vi "Read data.vi"(11 "communicator message in":refnum<class "communicator message.lvclass">) -> (3 "data":variant)   [LabVIEW 2015, in "communicator message.lvclass"]
uses:
  communicator message.lvclass
  communicator message.lvclass/communicator message.ctl
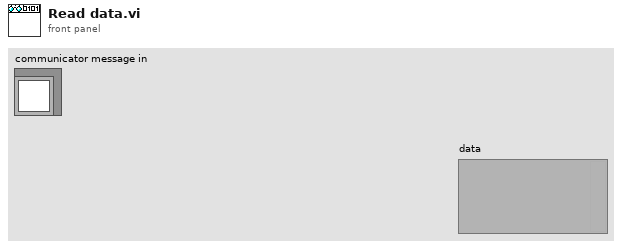
[diagram p1: front panel]
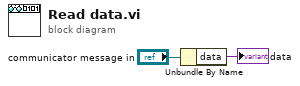
[diagram p0: block diagram]
diagram:
  n1 = Unbundle By Name("communicator message in") -> ("data"=→"data":variant)
